vi "Read endstop.vi"(7 "Simulate?":bool, 8 "error in (no error)":errorcluster, 11 "VISA Refnum in":refnum<visa-resource-name>) -> (0 "error out":errorcluster, 3 "Done?":bool)   [LabVIEW 2020, in "Monochromator.lvlib"]
uses:
  Monochromator.lvlib
  <vilib>/Instr/_visa.llb/VISA Flush IO Buffer Mask.ctl
panel:
  out "string":string
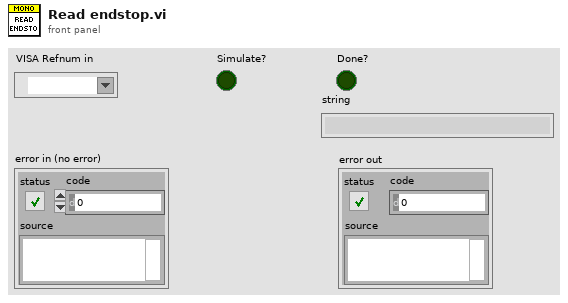
[diagram p1: front panel]
types:
  T1 = typedef "VISA Flush IO Buffer Mask.ctl" = u16
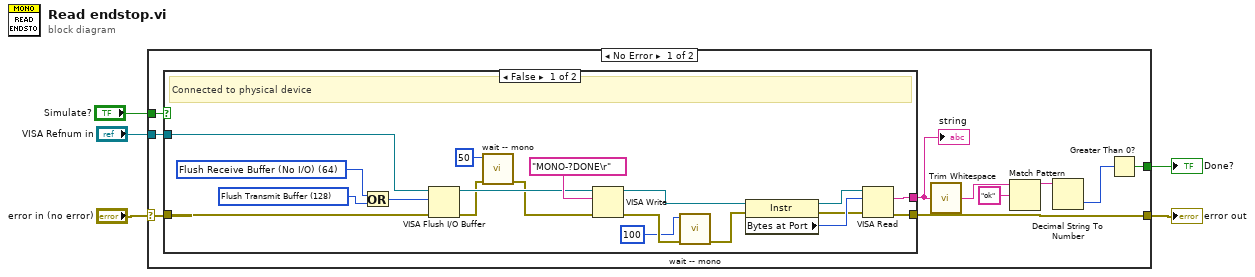
[diagram p0: block diagram]
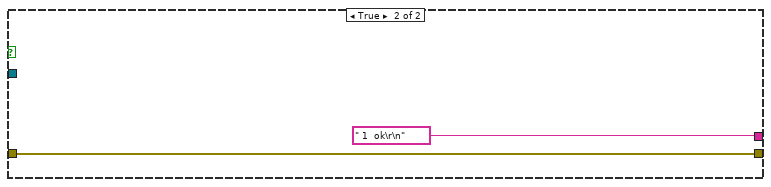
[diagram p2: hidden frame]
diagram:
  n1 = case shown="No Error" "error in (no error)" {
    selector: "error in (no error)" -> [w12 w37]
    tunnel: [w14 w37] -> w5
    tunnel: "VISA Refnum in" -> [w13 _]
    tunnel: [w10 _] -> w2
    tunnel: "Simulate?" -> [w6 _]
    frame No Error {
      n2 = case shown="False" w6 {
        tunnel: [w34 " 1  ok\r\n" ("string")] -> w15
        tunnel: [w33 w35] -> w14
        tunnel: w13 -> [w20 _]
        tunnel: w12 -> [w24 w35]
        frame False {
          w22 = T1 128 items=["Flush Receive Buffer"=16, "Write Transmit Buffer to Device"=32, "Flush Receive Buffer (No I/O)"=64, "Flush Transmit Buffer"=128] ("Mask")
          w23 = T1 64 items=["Flush Receive Buffer"=16, "Write Transmit Buffer to Device"=32, "Flush Receive Buffer (No I/O)"=64, "Flush Transmit Buffer"=128] ("Mask")
          # "Connected to physical device"
          n3 = Or(x=w23, y=w22) -> (x .or. y?=w21:T1)
          n4 = VISA Flush I/O Buffer(VISA resource name=w20, mask (16)=w21, error in (no error)=w24) -> (VISA resource name out=w19:refnum<visa-resource-name>, error out=w18:errorcluster)
          n5 = call "wait -- mono.vi"("error in (no error)"=w18, "milliseconds to wait"=u32 50) -> ("error out"=w17:errorcluster)  [unwired: 9 in]
          n6 = VISA Write(VISA resource name=w19, write buffer="MONO-?DONE\r" ("string"), error in (no error)=w17) -> (VISA resource name out=w29:refnum<visa-resource-name>, error out=w27:errorcluster)  [unwired: 1 out]
          n7 = call "wait -- mono.vi"("error in (no error)"=w27, "milliseconds to wait"=u32 100) -> ("error out"=w26:errorcluster)  [unwired: 9 in]
          n8 = property class="Instr"(reference=w29, error in=w26) -> (reference out=w31:refnum<visa-resource-name>, error out=w30:errorcluster, "Bytes at Port"=w32:u32)
          n9 = VISA Read(VISA resource name=w31, byte count=w32, error in (no error)=w30) -> (read buffer=w34:string, error out=w33:errorcluster)  [unwired: 2 out]
        }
        frame True {
        }
      }
      "string" <- w15
      n10 = call <vilib>:"Trim Whitespace.vi"("string"=w15) -> ("trimmed string"=w9:string)  [unwired: 1 in]
      n11 = Match Pattern(string=w9, regular expression="ok") -> (before substring=w8:string)  [unwired: 1 in, 3 out]
      n12 = Decimal String To Number(string=w8) -> (number=w11:i32)  [unwired: 2 in, 1 out]
      n13 = Greater Than 0?(x=w11) -> (x > 0?=w10:bool)
    }
    frame Error {
    }
  }
  "error out" <- w5
  "Done?" <- w2
